vi "disk_writeColumnHeadersAndTimeFormat.vi"(7 "column":T1, 8 "error in":errorcluster, 11 "DiskTemplate in":T4={"XMLRef"=[refnum, refnum, refnum, refnum, refnum, refnum], "ZipPath"=path "", "MetaFile"={"Ref"=refnum, "NextRow"=0, "NextPosition"=0, "Block"=[]}, "TempFolder"=path ""}) -> (0 "error out":errorcluster, 1 "styles map":string[](array[string]), 2 "formatted header length":i32, 3 "DiskTemplate out":T4)   [LabVIEW 2017, in "NI_ExcelFile.lvlib"]
uses:
  <vilib>/express/express shared/NI_ExcelFile/NI_ExcelFile.lvlib
  <vilib>/express/express shared/NI_ExcelFile/Ctrls/disk_TemplateFile.ctl
  <vilib>/express/express shared/NI_ExcelFile/Ctrls/meta_file.ctl
  <vilib>/express/express shared/NI_ExcelFile/Ctrls/meta_Block.ctl
  <vilib>/express/express shared/NI_ExcelFile/Ctrls/meta_BlockType.ctl
  <vilib>/express/express shared/NI_ExcelFile/Ctrls/Columns.ctl
  <vilib>/express/express shared/NI_ExcelFile/Ctrls/ColumnInfo.ctl
  <vilib>/express/express shared/NI_ExcelFile/Ctrls/DataType.ctl
  <vilib>/express/express shared/NI_ExcelFile/Ctrls/TemplateEnum.ctl
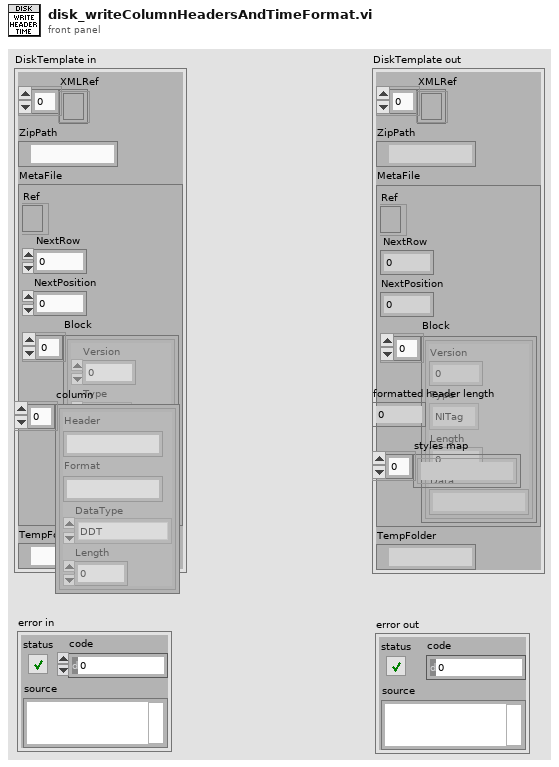
[diagram p1: front panel]
types:
  T1 = typedef "NI_ExcelFile.lvlib/Columns.ctl" = T2[]
  T2 = typedef "NI_ExcelFile.lvlib/ColumnInfo.ctl" = cluster{"Header":string, "Format":string, "DataType":T3, "Length":u64}
  T3 = typedef "NI_ExcelFile.lvlib/DataType.ctl" = enum16{"DDT", "WFM", "Array of STR", "Array of DBL", "Array of I8", "Array of I16", "Array of I32", "Array of I64", "Array of SGL", "Array of U8", "Array of U16", "Array of U32", "Array of U64", "Array of Time"}
  T4 = typedef "NI_ExcelFile.lvlib/disk_TemplateFile.ctl" = cluster{"XMLRef":refnum<file>[], "ZipPath":path, "MetaFile":T5, "TempFolder":path}
  T5 = typedef "NI_ExcelFile.lvlib/meta_file.ctl" = cluster{"Ref":refnum<file>, "NextRow":i32, "NextPosition":i64, "Block":T6[]}
  T6 = typedef "NI_ExcelFile.lvlib/meta_Block.ctl" = cluster{"Version":u16, "Type":T7, "Length":i32, "Data":string}
  T7 = typedef "NI_ExcelFile.lvlib/meta_BlockType.ctl" = enum16{"NITag", "File", "Column"}
  T8 = typedef "NI_ExcelFile.lvlib/TemplateEnum.ctl" = enum16{"[Content_Types].xml", ".rels", "workbook.xml", "styles.xml", "workbook.xml.rels", "sheet.xml", "app.xml", "core.xml"}
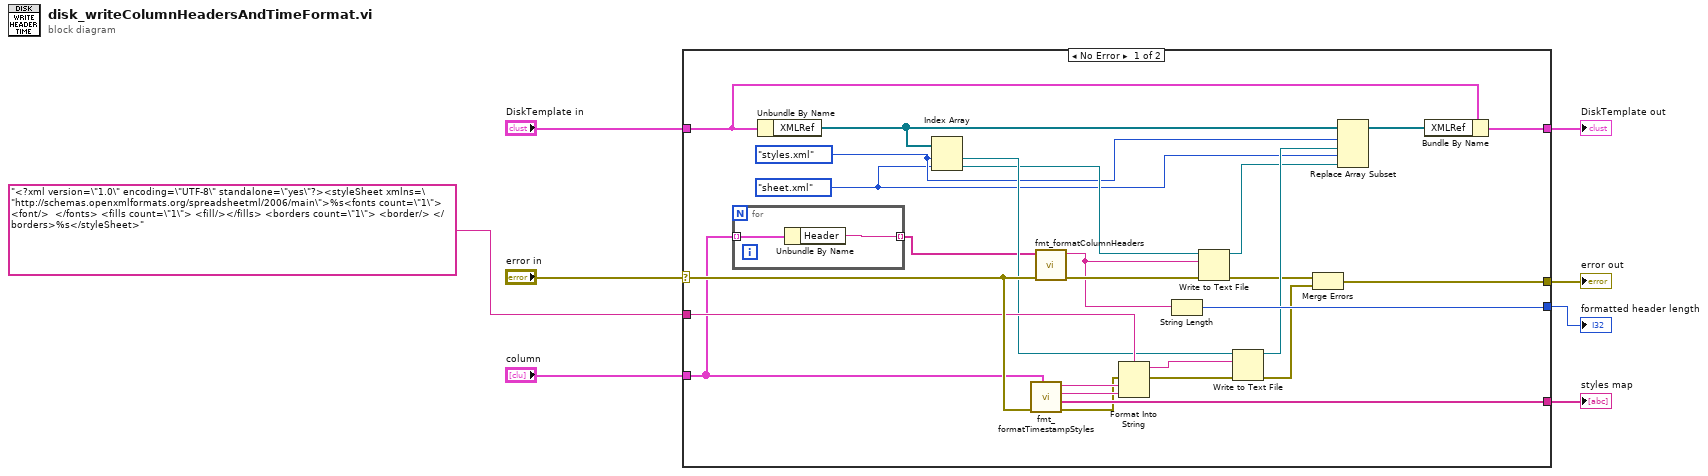
[diagram p0: block diagram]
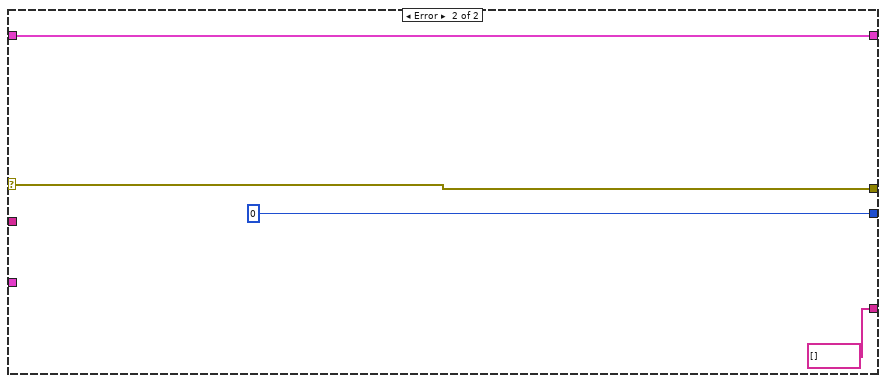
[diagram p2: hidden frame]
diagram:
  n1 = case shown="No Error" "error in" {
    selector: "error in" -> [w30 w39]
    tunnel: "DiskTemplate in" -> [w34 w40]
    tunnel: [w33 w40] -> w7
    tunnel: [w32 w39] -> w6
    tunnel: [w31 0] -> w5
    tunnel: "<?xml version=\"1.0\" encoding=\"UTF-8\" standalone=\"yes\"?><styleSheet xmlns=\"http://schemas.openxmlformats.org/spreadsheetml/2006/main\">%s<fonts count=\"1\">  <font/>  </fonts> <fills count=\"1\"> <fill/></fills> <borders count=\"1\"> <border/> </borders>%s</styleSheet>" ("string") -> [w29 _]
    tunnel: "column" -> [w12 _]
    tunnel: [w28 string[] [] ("time styles map")] -> w1
    frame No Error {
      w9 = TemplateEnum."sheet.xml" ("Template")
      w10 = TemplateEnum."styles.xml" ("Template")
      n2 = for {
        tunnel: w12 -> [w36] mode=indexing
        tunnel: [w35] -> w11 mode=indexing
        n3 = Unbundle By Name(w36) -> ("Header"=w35:string)
      }
      n4 = Unbundle By Name(w34) -> ("XMLRef"=w27:refnum<file>[])
      n5 = Index Array(array=w27, index #1=w10, index #2=w9) -> (element #1=w25:refnum<file>, element #2=w23:refnum<file>)
      n6 = call <vilib>:"fmt_formatTimestampStyles.vi"("Columns"=w12, "error in"=w30) -> ("error out"=w19:errorcluster, "styles map"=w28:string[], "cellXfs"=w20:string, "numFmts"=w21:string)  [unwired: 6 in]
      n7 = call <vilib>:"fmt_formatColumnHeaders.vi"("error in"=w30, "column headers"=w11) -> ("error out"=w18:errorcluster, "formatted column headers"=w17:string)  [unwired: 8 in]
      n8 = Format Into String(format string=w29, error in=w19, w21, w20) -> (resulting string=w16:string, error out=w15:errorcluster)  [unwired: 1 in]
      n9 = String Length(string=w17) -> (length=w31:i32)
      n10 = Write to Text File(file (use dialog)=w23, text=w17, error in=w18) -> (refnum out=w22:refnum<file>, error out=w14:errorcluster)  [unwired: 1 in, 1 out]
      n11 = Write to Text File(file (use dialog)=w25, text=w16, error in=w15) -> (refnum out=w24:refnum<file>, error out=w13:errorcluster)  [unwired: 1 in, 1 out]
      n12 = Merge Errors(w14, w13) -> (w32:errorcluster)
      n13 = Replace Array Subset(array=w27, new element #1=w24, index #1=w10, new element #2=w22, index #2=w9) -> (w26:refnum<file>[])
      n14 = Bundle By Name(cluster=w34, "XMLRef"=w26) -> (w33:T4)
    }
    frame Error {
    }
  }
  "DiskTemplate out" <- w7
  "error out" <- w6
  "formatted header length" <- w5
  "styles map" <- w1
